vi "SWERVE_DRIVE_MODULE_ACT.vi"(6 "Pass_Through_Time":dbl=-1.0 format="%33.4f", 8 "SwervePosInDeadband":bool=TRUE, 9 "Swerve State":T1={"Speed"=0.0, "Angle"={"VALUE"=0.0, "COS"=1.0, "SIN"=0.0}} {"Angle"."SIN" format="%13.4f"; "Angle"."COS" format="%13.4f"; "Angle"."VALUE" format="%13.4f"}, 10 "Swerve Dmd":T1={"Speed"=0.0, "Angle"={"VALUE"=0.0, "COS"=1.0, "SIN"=0.0}} {"Angle"."SIN" format="%13.4f"; "Angle"."COS" format="%13.4f"; "Angle"."VALUE" format="%13.4f"}, 11 "Swerve Module TypDef":T3) -> (0 "SwerveOnTarget":bool, 1 "SwervePosError":dbl, 2 "Swerve Motor Dmd":dbl, 3 "Wheel Motor Dmd":dbl, 4 "WheelSpeedErr":dbl)   [LabVIEW 2019]
uses:
  SWERVE_DRIVE_MODULE_TYPDEF.ctl
  <vilib>/Rock Robotics/WPI/MotorControl/WPI_MotorControlDeviceRef.ctl
  <vilib>/Rock Robotics/WPI/MotorControl/WPI_MotorControlType.ctl
  <vilib>/Rock Robotics/SystemInterfaces/DIO/FPGA_DIOPWMChannel.ctl
  <vilib>/Rock Robotics/WPI/PWM/WPI_PWMDeadband.ctl
  <vilib>/Rock Robotics/SystemInterfaces/DIO/FPGA_DIOChannel.ctl
  <vilib>/Rock Robotics/WPI/Encoder/WPI_EncoderDevRef.ctl
  <vilib>/Rock Robotics/SystemInterfaces/Encoder/FPGA_EncoderIdx.ctl
  <vilib>/Rock Robotics/SystemInterfaces/Counter/FPGA_CounterCtrSystemIndex.ctl
  <vilib>/Rock Robotics/WPI/Encoder/WPI_EncoderType.ctl
  <vilib>/Rock Robotics/WPI/ThirdParty/JAS_Junk/TrajLib/TypeDef/SWERVE_DRIVE_MODULE_STATE.ctl
  <vilib>/Rock Robotics/WPI/ThirdParty/JAS_Junk/TrajLib/TypeDef/ROTATION2D.ctl
  <vilib>/Rock Robotics/WPI/ThirdParty/JAS_Junk/TrajLib/TypeDef/X_Y_PAIR.ctl
  <vilib>/Rock Robotics/WPI/ThirdParty/JAS_Junk/TrajLib/VI/Util_GetTime_U32.vi
  <vilib>/Rock Robotics/WPI/ThirdParty/JAS_Junk/TrajLib/MathUtil_InputModulus.vi
  <vilib>/Rock Robotics/WPI/ThirdParty/JAS_Junk/TrajLib/Rotation2d_Minus.vi
  <vilib>/Rock Robotics/WPI/ThirdParty/JAS_Junk/TrajLib/Rotation2d_GetRadians.vi
  <vilib>/Rock Robotics/WPI/ThirdParty/JAS_Junk/TrajLib/SwerveModuleState_New.vi
  <vilib>/Rock Robotics/WPI/ThirdParty/JAS_Junk/TrajLib/Rotation2d_RotateBy.vi
  <vilib>/Rock Robotics/WPI/ThirdParty/JAS_Junk/TrajLib/Rotation2d_CreateAngle.vi
  <vilib>/Rock Robotics/WPI/ThirdParty/JAS_Junk/TrajLib/ProfiledPIDController_SetPID.vi
  <vilib>/Rock Robotics/WPI/ThirdParty/JAS_Junk/TrajLib/ProfiledPIDController_SetIntegratorRange.vi
  <vilib>/Rock Robotics/WPI/ThirdParty/JAS_Junk/TrajLib/ProfiledPIDController_SetTolerance_PosVel.vi
  <vilib>/Rock Robotics/WPI/ThirdParty/JAS_Junk/TrajLib/ProfiledPIDController_DisableContInput.vi
  <vilib>/Rock Robotics/WPI/ThirdParty/JAS_Junk/TrajLib/ProfiledPIDController_EnableContInput.vi
  <vilib>/Rock Robotics/WPI/ThirdParty/JAS_Junk/TrajLib/ProfiledPIDController_Reset_PosOnly.vi
  <vilib>/Rock Robotics/WPI/ThirdParty/JAS_Junk/TrajLib/ProfiledPIDController_NewPeriod.vi
  <vilib>/Rock Robotics/WPI/ThirdParty/JAS_Junk/TrajLib/ProfiledPIDController_Calculate_Meas_Goal.vi
  <vilib>/Rock Robotics/WPI/ThirdParty/JAS_Junk/TrajLib/ProfiledPIDController_AtGoal.vi
  <vilib>/Rock Robotics/WPI/ThirdParty/JAS_Junk/TrajLib/ProfiledPIDController_AtSetpoint.vi
  <vilib>/Rock Robotics/WPI/ThirdParty/JAS_Junk/TrajLib/ProfiledPIDController_SetConstraints.vi
  <vilib>/Rock Robotics/WPI/ThirdParty/JAS_Junk/TrajLib/VI/FunctionGenerator_New.vi
  <vilib>/Rock Robotics/WPI/ThirdParty/JAS_Junk/TrajLib/VI/FunctionGenerator_Calculate.vi
  <vilib>/Rock Robotics/WPI/ThirdParty/JAS_Junk/TrajLib/PIDController_AtSetpoint.vi
  <vilib>/Rock Robotics/WPI/ThirdParty/JAS_Junk/TrajLib/PIDController_SetPIDF.vi
  <vilib>/Rock Robotics/WPI/ThirdParty/JAS_Junk/TrajLib/PIDController_SetDerivativeFilter.vi
  <vilib>/Rock Robotics/WPI/ThirdParty/JAS_Junk/TrajLib/PIDController_SetIntegratorRange.vi
  <vilib>/Rock Robotics/WPI/ThirdParty/JAS_Junk/TrajLib/PIDController_SetTolerancePandV.vi
  <vilib>/Rock Robotics/WPI/ThirdParty/JAS_Junk/TrajLib/PIDController_DisableContinousInput.vi
  <vilib>/Rock Robotics/WPI/ThirdParty/JAS_Junk/TrajLib/PIDController_EnableContinousInput.vi
  <vilib>/Rock Robotics/WPI/ThirdParty/JAS_Junk/TrajLib/PIDController_Reset.vi
  <vilib>/Rock Robotics/WPI/ThirdParty/JAS_Junk/TrajLib/PIDController_New.vi
  <vilib>/Rock Robotics/WPI/ThirdParty/JAS_Junk/TrajLib/PIDController_SetOutputLimits.vi
  <vilib>/Rock Robotics/WPI/ThirdParty/JAS_Junk/TrajLib/SlewRateLimiter_New.vi
  <vilib>/Rock Robotics/WPI/ThirdParty/JAS_Junk/TrajLib/SlewRateLimiter_Reset.vi
  <vilib>/Rock Robotics/WPI/ThirdParty/JAS_Junk/TrajLib/SlewRateLimiter_Calculate.vi
  <vilib>/Rock Robotics/WPI/ThirdParty/JAS_Junk/TrajLib/SlewRateLimiter_SetRate.vi
  <vilib>/Rock Robotics/WPI/ThirdParty/JAS_Junk/TrajLib/Rotation2d_UnaryMinus.vi
  <vilib>/Rock Robotics/WPI/ThirdParty/JAS_Junk/TrajLib/Rotation2d_CreateXY.vi
  <vilib>/Rock Robotics/WPI/ThirdParty/JAS_Junk/TrajLib/PIDController_SetPID.vi
  <vilib>/Rock Robotics/WPI/ThirdParty/JAS_Junk/TrajLib/TrapProfState_New.vi
  <vilib>/Rock Robotics/WPI/ThirdParty/JAS_Junk/TrajLib/ProfiledPIDController_Reset.vi
  <vilib>/Rock Robotics/WPI/ThirdParty/JAS_Junk/TrajLib/PIDController_NewPeriod.vi
  <vilib>/Rock Robotics/SystemInterfaces/NetworkCommunication/NetComm_UsageReport_report.vi
  <vilib>/Rock Robotics/WPI/ThirdParty/JAS_Junk/TrajLib/ProfiledPIDController_SetGoal_PosOnly.vi
  <vilib>/Rock Robotics/WPI/ThirdParty/JAS_Junk/TrajLib/ProfiledPIDController_Calculate_Meas.vi
  <vilib>/Rock Robotics/WPI/ThirdParty/JAS_Junk/TrajLib/TrapProfState_Equals.vi
  <vilib>/Rock Robotics/WPI/ThirdParty/JAS_Junk/TrajLib/Util_CalcDist.vi
  <vilib>/Rock Robotics/WPI/ThirdParty/JAS_Junk/TrajLib/ProfiledPIDController_SetGoal.vi
  <vilib>/Rock Robotics/WPI/ThirdParty/JAS_Junk/TrajLib/PIDController_Calculate_SP_PV.vi
  <vilib>/Rock Robotics/WPI/ThirdParty/JAS_Junk/TrajLib/TrapProfile_New.vi
  <vilib>/Rock Robotics/WPI/ThirdParty/JAS_Junk/TrajLib/ProfiledPIDController_GetPeriod.vi
  <vilib>/Rock Robotics/WPI/ThirdParty/JAS_Junk/TrajLib/TrapProfile_Calculate.vi
  <vilib>/Rock Robotics/WPI/ThirdParty/JAS_Junk/TrajLib/ControllerUtil_GetModulusError.vi
  <vilib>/Rock Robotics/WPI/ThirdParty/JAS_Junk/TrajLib/PIDController_SetSetpoint.vi
  <vilib>/Rock Robotics/WPI/ThirdParty/JAS_Junk/TrajLib/PIDController_Calculate_PV.vi
  <vilib>/Rock Robotics/WPI/ThirdParty/JAS_Junk/TrajLib/TrapProfile_ShouldFlipAcceleration.vi
  <vilib>/Rock Robotics/WPI/ThirdParty/JAS_Junk/TrajLib/TrapProfile_Direct.vi
  <vilib>/Rock Robotics/WPI/ThirdParty/JAS_Junk/TrajLib/PIDController_GetPeriod.vi
  <vilib>/gmath/interp.llb/Search Ordered Table.vi
  <vilib>/Rock Robotics/WPI/ThirdParty/JAS_Junk/TrajLib/VI/Util_GetTime_U64.vi
  <vilib>/Rock Robotics/WPI/ThirdParty/JAS_Junk/TrajLib/Globals/Util_LibraryGlobals.vi
  <vilib>/Rock Robotics/WPI/ThirdParty/JAS_Junk/TrajLib/PIDController_AdvCalculate_FF_Sp_Pv.vi
  <vilib>/Rock Robotics/WPI/ThirdParty/JAS_Junk/TrajLib/Trajectory_Library.lvlib
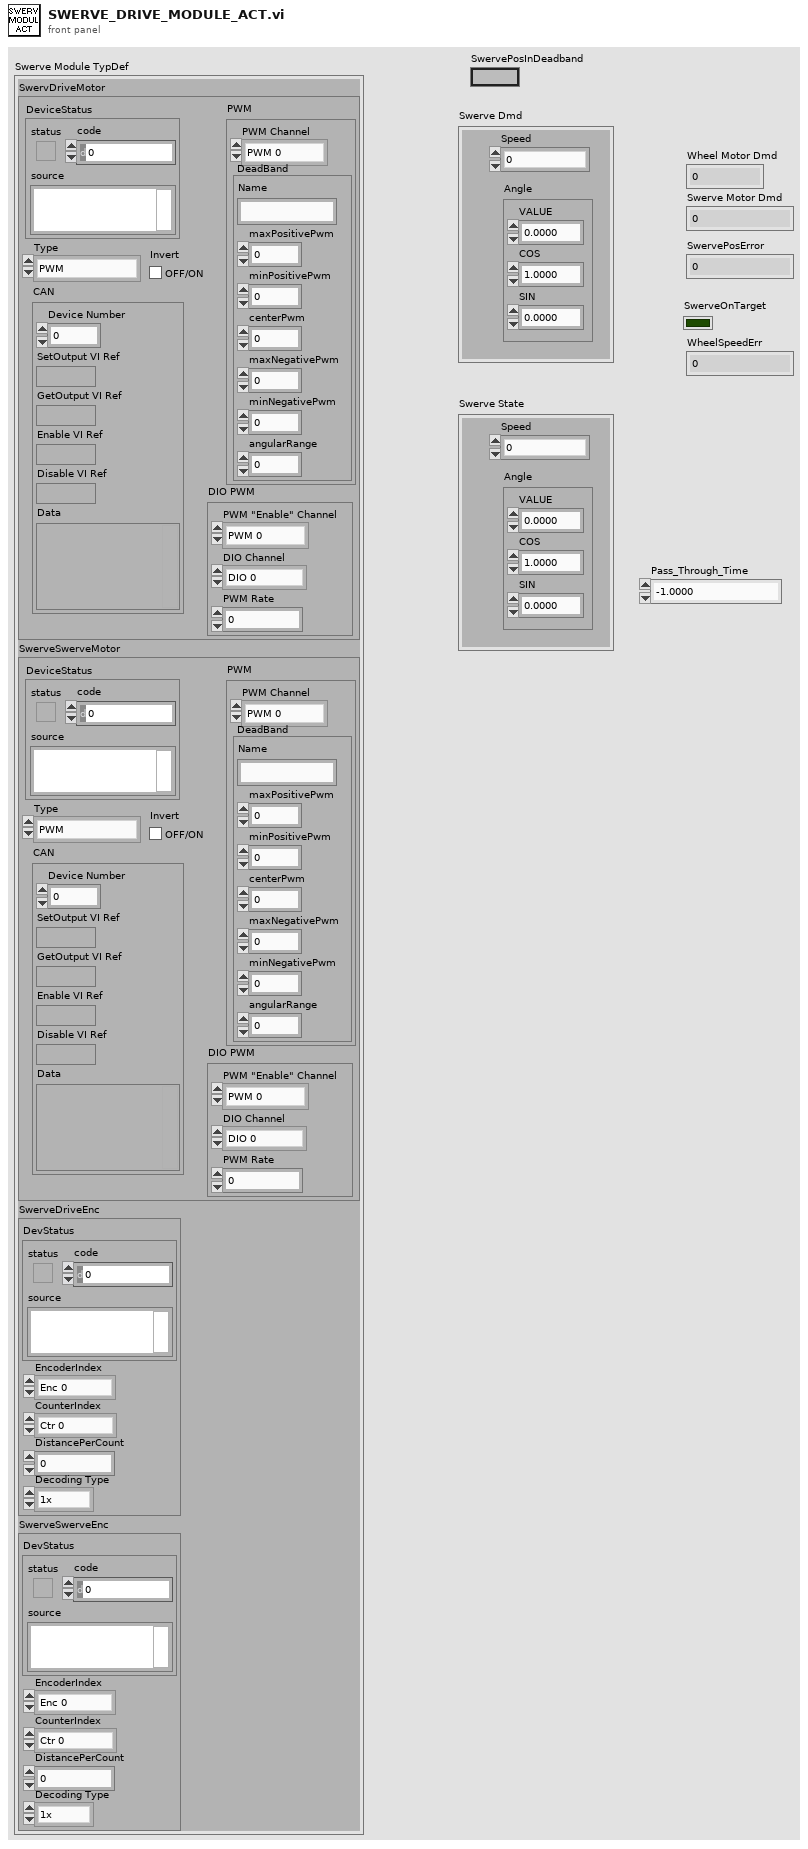
[diagram p1: front panel]
types:
  T1 = typedef "Trajectory_Library.lvlib/SWERVE_DRIVE_MODULE_STATE.ctl" = cluster{"Speed":dbl, "Angle":T2}
  T2 = typedef "Trajectory_Library.lvlib/ROTATION2D.ctl" = cluster{"VALUE":dbl, "COS":dbl, "SIN":dbl}
  T3 = typedef "SWERVE_DRIVE_MODULE_TYPDEF.ctl" = cluster{"SwervDriveMotor":T4, "SwerveSwerveMotor":T4, "SwerveDriveEnc":T9, "SwerveSwerveEnc":T9}
  T4 = typedef "WPI_MotorControlDeviceRef.ctl" = cluster{"DeviceStatus":errorcluster, "Type":T5, "PWM":cluster{"PWM Channel":T6, "DeadBand":T7}, "CAN":cluster{"Device Number":u8, "SetOutput VI Ref":variant, "GetOutput VI Ref":variant, "Enable VI Ref":variant, "Disable VI Ref":variant, "Data":variant}, "Invert":bool, "DIO PWM":cluster{"PWM \"Enable\" Channel":T6, "DIOChannel":T8, "PWM Rate":dbl}}
  T5 = typedef "WPI_MotorControlType.ctl" = enum16{"PWM", "CAN", "DIO PWM"}
  T6 = typedef "FPGA_DIOPWMChannel.ctl" = enum8{"PWM 0", "PWM 1", "PWM 2", "PWM 3", "PWM 4", "PWM 5", "PWM 6", "PWM 7", "PWM 8", "PWM 9", "PWM MXP 0", "PWM MXP 1", "PWM MXP 2", "PWM MXP 3", "PWM MXP 4", "PWM MXP 5", "PWM MXP 6", "PWM MXP 7", "PWM MXP 8", "PWM MXP 9", "Invalid"}
  T7 = typedef "WPI_PWMDeadband.ctl" = cluster{"Name":string, "maxPositivePwm":i32, "minPositivePwm":i32, "centerPwm":i32, "maxNegativePwm":i32, "minNegativePwm":i32, "angularRange":u16}
  T8 = typedef "FPGA_DIOChannel.ctl" = enum8{"DIO 0", "DIO 1", "DIO 2", "DIO 3", "DIO 4", "DIO 5", "DIO 6", "DIO 7", "DIO 8", "DIO 9", "DIO MXP 0", "DIO MXP 1", "DIO MXP 2", "DIO MXP 3", "DIO MXP 4", "DIO MXP 5", "DIO MXP 6", "DIO MXP 7", "DIO MXP 8", "DIO MXP 9", "DIO MXP 10", "DIO MXP 11", "DIO MXP 12", "DIO MXP 13", "DIO MXP 14", "DIO MXP 15", "SPI Port CS1", "SPI Port CS2", "SPI Port CS3", "SPI Port MISO", "SPI Port MOSI", "Invalid"}
  T9 = typedef "WPI_EncoderDevRef.ctl" = cluster{"DevStatus":errorcluster, "EncoderIndex":T10, "CounterIndex":T11, "DistancePerCount":dbl, "Decoding Type":T12}
  T10 = typedef "FPGA_EncoderIdx.ctl" = enum8{"Enc 0", "Enc 1", "Enc 2", "Enc 3", "Enc 4", "Enc 5", "Enc 6", "Enc 7", "Invalid"}
  T11 = typedef "FPGA_CounterCtrSystemIndex.ctl" = enum8{"Ctr 0", "Ctr 1", "Ctr 2", "Ctr 3", "Ctr 4", "Ctr 5", "Ctr 6", "Ctr 7", "Invalid"}
  T12 = typedef "WPI_EncoderType.ctl" = enum16{"1x", "2x", "4x"}
  T13 = typedef "Trajectory_Library.lvlib/X_Y_PAIR.ctl" = cluster{"X":dbl, "Y":dbl}
  T14 = typedef "Trajectory_Library.lvlib/PID_TUNING.ctl" = cluster{"Kp":dbl, "Ki":dbl, "Kd":dbl, "MaximumIntegral":dbl, "MinimumIntegral":dbl}
  T15 = typedef "Trajectory_Library.lvlib/PID_ERROR_TOLERANCE.ctl" = cluster{"PositionTolerance":dbl, "VelocityTolerance":dbl}
  T16 = typedef "Trajectory_Library.lvlib/PID_INPUT_LIMITS.ctl" = cluster{"MaxInput":dbl, "MinInput":dbl, "Continuous":bool}
  T17 = typedef "Trajectory_Library.lvlib/TRAPEZOID_PROFILE_CONSTRAINT.ctl" = cluster{"MaxVelocity":dbl, "MaxAcceleration":dbl}
  T18 = typedef "Trajectory_Library.lvlib/PID_ADV_LIMITS.ctl" = cluster{"MaxInput":dbl, "MinInput":dbl, "Continuous":bool, "MaxOutput":dbl, "MinOutput":dbl}
  T19 = typedef "Trajectory_Library.lvlib/PID_ADV_TUNING.ctl" = cluster{"Kf":dbl, "Kp":dbl, "Ki":dbl, "Kd":dbl, "MaximumIntegral":dbl, "MinimumIntegral":dbl, "Filter Derivative":bool}
  T20 = typedef "Trajectory_Library.lvlib/PID_CONTROLLER.ctl" = cluster{"Kp":dbl, "Ki":dbl, "Kd":dbl, "Period":dbl, "Max_Integral":dbl, "Min_Integral":dbl, "Max_Input":dbl, "Min_Input":dbl, "Continuous":bool, "PositionError":dbl, "VelocityError":dbl, "PrevError":dbl, "TotalError":dbl, "PositionTolerance":dbl, "VelocityTolerance":dbl, "SetPoint":dbl, "Kf":dbl, "Prev_Deriv":dbl, "Prev_Deriv 2":dbl, "DerivativeFilter":bool, "Min_Output":dbl, "Max_Output":dbl, "Prev_F_P":dbl, "Prev_F_P_2":dbl, "AntiWindupActive":bool, "Measurement":dbl}
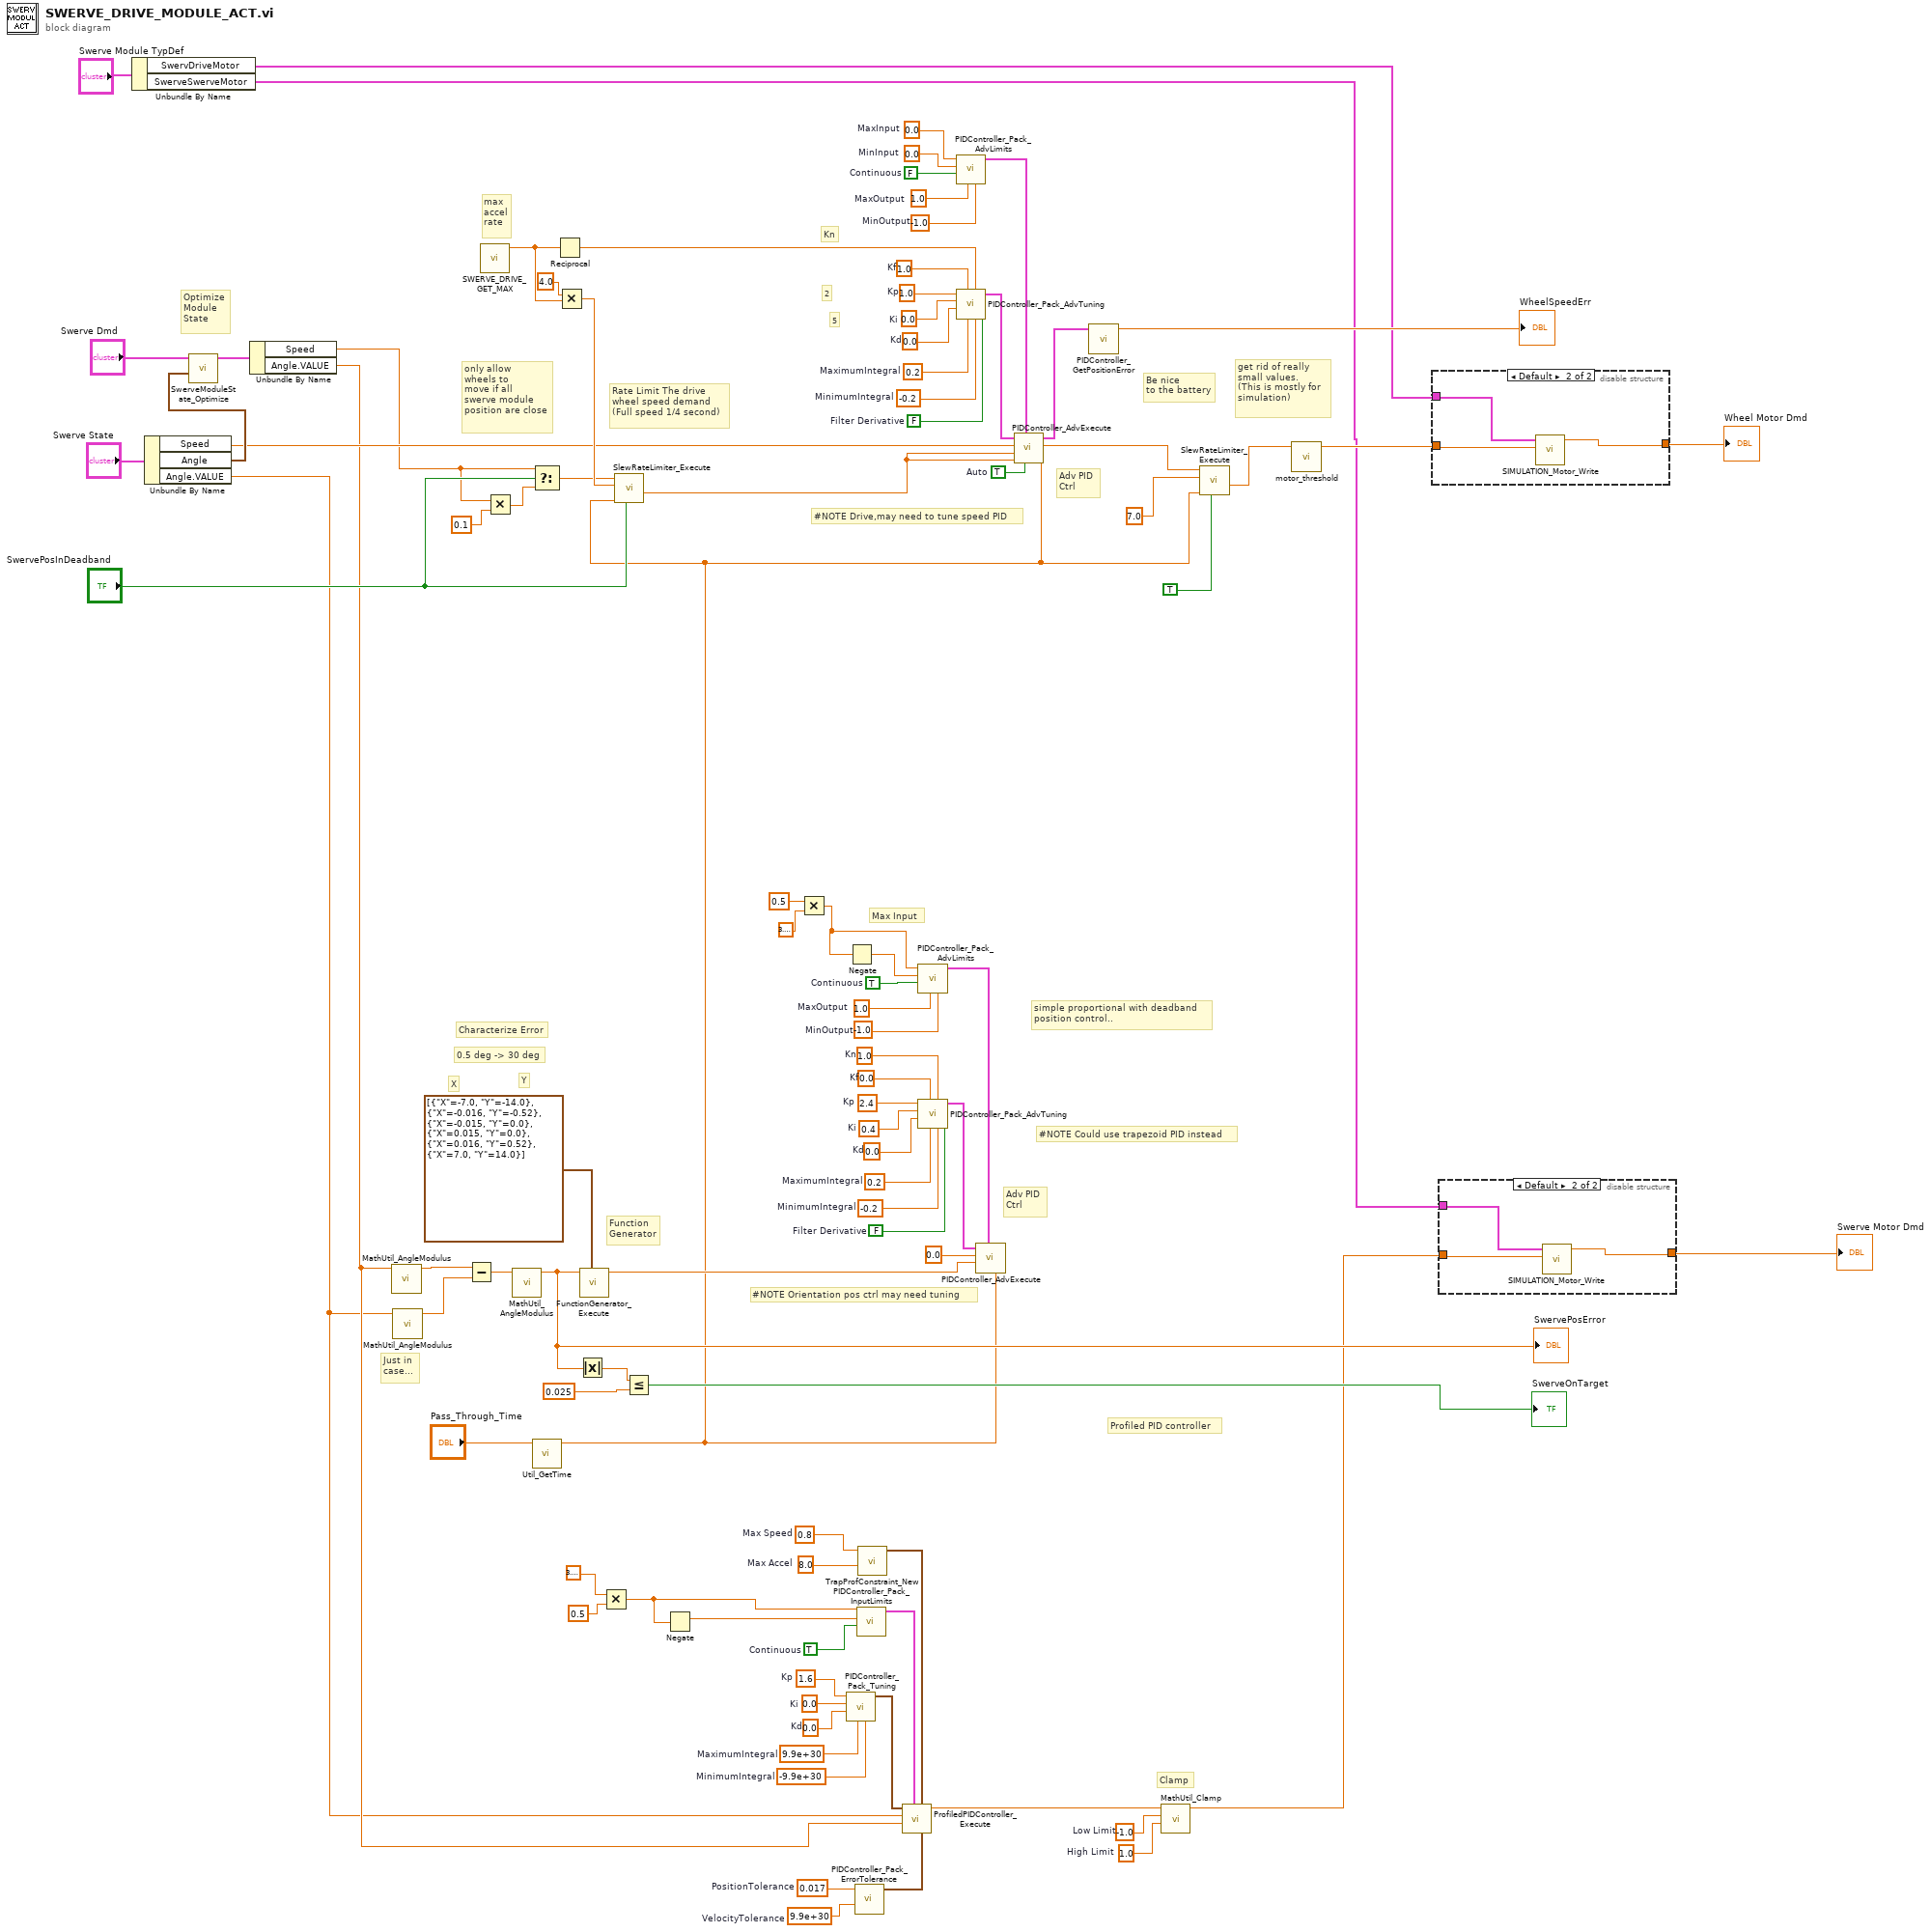
[diagram p0: block diagram]
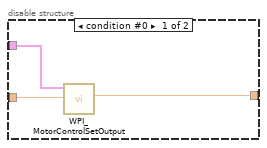
[diagram p2: hidden frame]
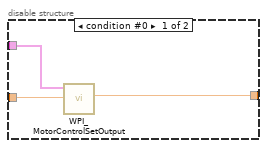
[diagram p3: hidden frame]
diagram:
  w7 = 1.0  # High Limit
  w6 = -1.0  # Low Limit
  w35 = 0.017  # PositionTolerance
  w34 = 9.9e+30  # VelocityTolerance
  w32 = 0.8  # Max Speed
  w31 = 8.0  # Max Accel
  w29 = TRUE  # Continuous
  w28 = 1.6  # Kp
  w27 = 0.0  # Ki
  w26 = 0.0  # Kd
  w25 = 9.9e+30  # MaximumIntegral
  w24 = -9.9e+30  # MinimumIntegral
  w44 = TRUE  # Auto
  w60 = 1.0  # Kp
  w59 = 0.0  # Ki
  w58 = 0.0  # Kd
  w57 = 1.0  # Kf
  w56 = 0.2  # MaximumIntegral
  w55 = -0.2  # MinimumIntegral
  w54 = FALSE  # Filter Derivative
  w52 = 0.0  # MinInput
  w51 = FALSE  # Continuous
  w50 = 1.0  # MaxOutput
  w53 = -1.0  # MinOutput
  w49 = 0.0  # MaxInput
  w73 = 1.0  # MaxOutput
  w74 = -1.0  # MinOutput
  w88 = 1.0  # Kn
  w87 = 2.4  # Kp
  w86 = 0.4  # Ki
  w85 = 0.0  # Kd
  w84 = 0.0  # Kf
  w83 = 0.2  # MaximumIntegral
  w82 = -0.2  # MinimumIntegral
  w81 = FALSE  # Filter Derivative
  w80 = TRUE  # Continuous
  # "Clamp"
  # "Be nice\nto the battery"
  # "5"
  # "2"
  # "Profiled PID controller"
  # "Optimize\nModule\nState"
  # "Kn"
  # "Adv PID\nCtrl"
  # "Rate Limit The drive\nwheel speed demand\n(Full speed 1/4 second)"
  # "Just in \ncase..."
  # "#NOTE Could use trapezoid PID instead"
  # "Characterize Error"
  # "Max Input"
  # "Adv PID\nCtrl"
  # "0.5 deg -> 30 deg"
  # "Function\nGenerator"
  # "Y"
  # "X"
  # "#NOTE Orientation pos ctrl may need tuning"
  # "only allow\nwheels to \nmove if all \nswerve module \nposition are close"
  # "#NOTE Drive,may need to tune speed PID"
  # "simple proportional with deadband\nposition control.."
  # "get rid of really\nsmall values.\n(This is mostly for \nsimulation)"
  # "max\naccel\nrate"
  n1 = Unbundle By Name("Swerve Module TypDef") -> ("SwervDriveMotor"=w40:T4, "SwerveSwerveMotor"=w38:T4)
  n2 = Unbundle By Name("Swerve State") -> ("Speed"=w45:dbl, "Angle"=w63:T2, "Angle.VALUE"=w19:dbl)
  n3 = call <vilib>:"SwerveModuleState_Optimize.vi"("CurrentAngle"=w63, "Desired State"="Swerve Dmd") -> ("out SWERVE_DRIVE_MODULE_STATE"=w62:T1)  [unwired: 9 in]
  n4 = Unbundle By Name(w62) -> ("Speed"=w13:dbl, "Angle.VALUE"=w20:dbl)
  n5 = call <vilib>:"MathUtil_AngleModulus.vi"("InputAngle"=w20) -> ("ModulsAngle"=w68:dbl)  [unwired: 10 in]
  n6 = call <vilib>:"MathUtil_AngleModulus.vi"("InputAngle"=w19) -> ("ModulsAngle"=w67:dbl)  [unwired: 10 in]
  n7 = Subtract(x=w68, y=w67) -> (x-y=w69:dbl)
  n8 = call "SWERVE_DRIVE_GET_MAX.vi"() -> ("Max Wheel Vel (Meter/Sec)"=w93:dbl)  [unwired: 10 in, 1 out]
  n9 = Multiply(x=w13, y=0.1) -> (x*y=w11:dbl)
  n10 = call <vilib>:"MathUtil_AngleModulus.vi"("InputAngle"=w69) -> ("ModulsAngle"=w66:dbl)  [unwired: 10 in]
  "SwervePosError" <- w66
  n11 = Select(t=w13, s="SwervePosInDeadband", f=w11) -> (s? t:f=w90:dbl)
  n12 = call <vilib>:"Util_GetTime.vi"("Pass_Through_Time"="Pass_Through_Time") -> ("FPGA_Time_Seconds"=w15:dbl)  [unwired: 8 in, 2 out]
  n13 = Reciprocal(x=w93) -> (1/x=w46:dbl)
  n14 = Multiply(x=4.0, y=w93) -> (x*y=w91:dbl)
  n15 = Absolute Value(x=w66) -> (abs(x)=w72:dbl)
  n16 = call <vilib>:"FunctionGenerator_Execute.vi"("X Y Pairs"=T13[] [{"X"=-7.0, "Y"=-14.0}, {"X"=-0.016, "Y"=-0.52}, {"X"=-0.015, "Y"=0.0}, {"X"=0.015, "Y"=0.0}, {"X"=0.016, "Y"=0.52}, {"X"=7.0, "Y"=14.0}], "Input Value"=w66) -> ("Output Value"=w75:dbl)  [unwired: 9 in]
  n17 = Multiply(x=3.141592653589793, y=0.5) -> (x*y=w1:dbl)
  n18 = call <vilib>:"SlewRateLimiter_Execute.vi"("Enable"="SwervePosInDeadband", "Time"=w15, "PositiveRate"=w91, "Input"=w90) -> ("Output"=w41:dbl)  [unwired: 6 in, 1 out]
  n19 = Less Or Equal?(x=w72, y=0.025 ("ErrDeadband")) -> (x <= y?=→"SwerveOnTarget":bool)
  n20 = Negate(x=w1) -> (-x=w21:dbl)
  n21 = Multiply(x=0.5, y=3.141592653589793) -> (x*y=w10:dbl)
  n22 = call <vilib>:"PIDController_Pack_Tuning.vi"("MinimumIntegral"=w24, "MaximumIntegral"=w25, "Kd"=w26, "Ki"=w27, "Kp"=w28) -> ("PID Tuning"=w23:T14)  [unwired: 6 in]
  n23 = Negate(x=w10) -> (-x=w77:dbl)
  n24 = call <vilib>:"PIDController_Pack_ErrorTolerance.vi"("VelocityTolerance"=w34, "PositionTolerance"=w35) -> ("PID Error Tolerance"=w33:T15)  [unwired: 9 in]
  n25 = call <vilib>:"PIDController_Pack_InputLimits.vi"("Continuous"=w29, "MinInput"=w21, "MaxInput"=w1) -> ("PID Input Limits"=w22:T16)  [unwired: 8 in]
  n26 = call <vilib>:"TrapProfConstraint_New.vi"("Max Accel"=w31, "Max Speed (M/S)"=w32) -> ("TRAPEZOID_PROFILE_CONSTRAINT"=w30:T17)  [unwired: 9 in]
  n27 = call <vilib>:"ProfiledPIDController_Execute.vi"("PID Error Tolerance"=w33, "Constraints"=w30, "PID Input Limits"=w22, "SP-SetPoint Goal"=w20, "PV-Measurement"=w19, "PID Tuning"=w23) -> ("CO-ControlOutput"=w5:dbl)  [unwired: 2 in, 3 out]
  n28 = call <vilib>:"PIDController_Pack_AdvLimits.vi"("MinOutput"=w74, "MaxOutput"=w73, "Continuous"=w80, "MinInput"=w77, "MaxInput"=w10) -> ("Adv PID Limits"=w78:T18)  [unwired: 6 in]
  n29 = call <vilib>:"PIDController_Pack_AdvTuning.vi"("Filter Derivative"=w81, "MinimumIntegral"=w82, "Kn"=w88, "MaximumIntegral"=w83, "Kf"=w84, "Kd"=w85, "Ki"=w86, "Kp"=w87) -> ("Adv PID Tuning"=w79:T19)  [unwired: 3 in]
  n30 = call <vilib>:"PIDController_Pack_AdvLimits.vi"("MinOutput"=w53, "MaxOutput"=w50, "Continuous"=w51, "MinInput"=w52, "MaxInput"=w49) -> ("Adv PID Limits"=w47:T18)  [unwired: 6 in]
  n31 = call <vilib>:"PIDController_Pack_AdvTuning.vi"("Filter Derivative"=w54, "MinimumIntegral"=w55, "Kn"=w46, "MaximumIntegral"=w56, "Kf"=w57, "Kd"=w58, "Ki"=w59, "Kp"=w60) -> ("Adv PID Tuning"=w48:T19)  [unwired: 3 in]
  n32 = call <vilib>:"PIDController_AdvExecute.vi"("Time"=w15, "Adv PID Limits"=w78, "SP-SetPoint"=w75, "PV-Measurement"=0.0, "Adv PID Tuning"=w79) -> ()  [unwired: 4 in, 3 out]
  n33 = call <vilib>:"PIDController_AdvExecute.vi"("Time"=w15, "Auto"=w44, "Adv PID Limits"=w47, "FF-FeedForward"=w41, "SP-SetPoint"=w41, "PV-Measurement"=w45, "Adv PID Tuning"=w48) -> ("CO-ControlOutput"=w18:dbl, "out PID_CONTROLLER"=w43:T20)  [unwired: 2 in, 1 out]
  n34 = call <vilib>:"PIDController_GetPositionError.vi"("in PID_CONTROLLER"=w43) -> ("PositionError"=→"WheelSpeedErr":dbl)  [unwired: 10 in]
  n35 = call <vilib>:"MathUtil_Clamp.vi"("High Limit"=w7, "Low Limit"=w6, "Value"=w5) -> ("Result"=w4:dbl)  [unwired: 8 in]
  n36 = call <vilib>:"SlewRateLimiter_Execute.vi"("Enable"=TRUE, "Time"=w15, "PositiveRate"=7.0, "Input"=w18) -> ("Output"=w17:dbl)  [unwired: 6 in, 1 out]
  n37 = call "motor_threshold.vi"("motor in"=w17) -> ("motor out"=w39:dbl)  [unwired: 10 in]
  n38 = disable-structure shown="Default" {
    disable-tunnel: w39 -> [w98 w100]
    disable-tunnel: w40 -> [w97 w101]
    disable-tunnel: [w96 w99] -> w37
    frame condition #0 {
      n39 = call <vilib>:"WPI_MotorControlSetOutput.vi"("Output"=w98, "MotorControlDevRef"=w97) -> ("Motor Output"=w96:dbl)  [unwired: 7 in, 2 out]
    }
    frame condition #1 (active) {
      n40 = call "SIMULATION_Motor_Write.vi"("Motor Demand"=w100, "Motor Device Reference"=w101) -> ("Out Motor Demand"=w99:dbl)  [unwired: 9 in]
    }
  }
  "Wheel Motor Dmd" <- w37
  n41 = disable-structure shown="Default" {
    disable-tunnel: w4 -> [w104 w106]
    disable-tunnel: w38 -> [w103 w107]
    disable-tunnel: [w102 w105] -> w36
    frame condition #0 {
      n42 = call <vilib>:"WPI_MotorControlSetOutput.vi"("Output"=w104, "MotorControlDevRef"=w103) -> ("Motor Output"=w102:dbl)  [unwired: 7 in, 2 out]
    }
    frame condition #1 (active) {
      n43 = call "SIMULATION_Motor_Write.vi"("Motor Demand"=w106, "Motor Device Reference"=w107) -> ("Out Motor Demand"=w105:dbl)  [unwired: 9 in]
    }
  }
  "Swerve Motor Dmd" <- w36
